vi "Startup.vi"(6 "LabVIEW Web Service":refnum<class "Web Service.lvclass">) -> ()   [LabVIEW 2014]
uses:
  <vilib>/wsapi/Web Service.lvclass
  Configuration/Global_Configurations.vi
panel:
  # "Use the web service input terminal to call the VIs on the Service subpalette of the Web Services palette. Do not remove it from the connector pane unless you don't need access to the palette."
  # "Any additional terminals added to the connector pane of a startup VI will be ignored."
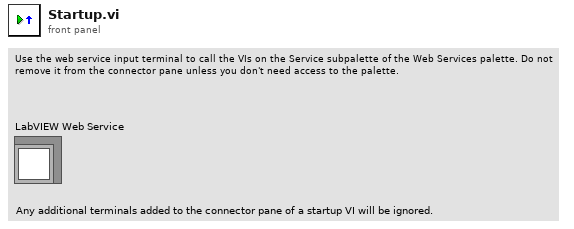
[diagram p1: front panel]
types:
  T1 = cluster{"Path":path, "Name":string, "Authors":string, "Keywords":string, "Description":string, "Cameras":cluster{"Base URL":string, "Path":string, "Name":string}[]}[]
  T2 = cluster{"Path":path, "Name":string, "Authors":string, "Keywords":string, "Description":string, "Cameras":cluster{"Base URL":string, "Path":string, "Name":string}[]}
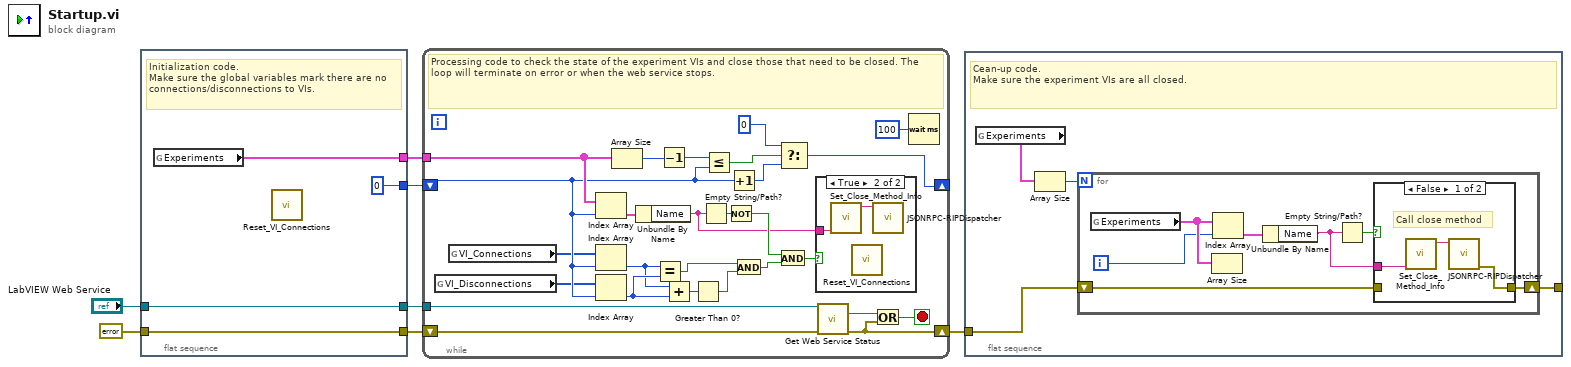
[diagram p0: block diagram]
diagram:
  n1 = flat-sequence {
    tunnel: "LabVIEW Web Service" -> [w11]
    tunnel: [w11] -> w6
    tunnel: [w10] -> w5
    tunnel: errorcluster {"status"=FALSE, "code"=0, "source"=""} ("error constant") -> [w10]
    tunnel: [0] -> w2
    tunnel: [w8] -> w1
    frame #0 {
      # "Initialization code.\nMake sure the global variables mark there are no connections/disconnections to VIs."
      n2 = global read "Global_Configurations.vi" "Experiments"() -> (w8:T1)
      n3 = call "Reset_VI_Connections.vi"() -> ()  [unwired: 12 in]
    }
  }
  n4 = while {
    tunnel: w6 -> [w37]
    shift-right: [w34] -> w3
    shift-left: w5 -> [w35]
    shift-right: [w25] -> _
    shift-left: w2 -> [w20]
    tunnel: w1 -> [w22]
    stop <- w36 stop-if-true
    # "Processing code to check the state of the experiment VIs and close those that need to be closed. The loop will terminate on error or when the web service stops."
    n5 = global read "Global_Configurations.vi" "VI_Disconnections"() -> (w14:u8[])
    n6 = global read "Global_Configurations.vi" "VI_Connections"() -> (w15:u8[])
    n7 = Index Array(array=w22, index=w20) -> (element=w29:T2)
    n8 = Index Array(array=w15, index=w20) -> (element=w12:u8)
    n9 = Index Array(array=w14, index=w20) -> (element=w13:u8)
    n10 = Array Size(array=w22) -> (size(s)=w28:i32)
    n11 = Unbundle By Name(w29) -> ("Name"=w21:string)
    n12 = Equal?(x=w12, y=w13) -> (x = y?=w18:bool)
    n13 = Decrement(x=w28) -> (x-1=w27:i32)
    n14 = Add(x=w12, y=w13) -> (x+y=w16:u8)
    n15 = Greater Than 0?(x=w16) -> (x > 0?=w17:bool)
    n16 = Empty String/Path?(string/path=w21) -> (empty?=w30:bool)
    n17 = Less Or Equal?(x=w27, y=w20) -> (x <= y?=w26:bool)
    n18 = Not(x=w30) -> (.not. x?=w31:bool)
    n19 = Increment(x=w20) -> (x+1=w23:i32)
    n20 = And(x=w18, y=w17) -> (x .and. y?=w19:bool)
    n21 = And(x=w31, y=w19) -> (x .and. y?=w32:bool)
    n22 = Select(t=0 ("f"), s=w26, f=w23) -> (s? t:f=w25:i32)
    n23 = case shown="True" w32 {
      tunnel: w21 -> [_ w39]
      frame False {
      }
      frame True {
        n24 = call "Set_Close_Method_Info.vi"("expId"=w39) -> ("String"=w40:string)  [unwired: 10 in]
        n25 = call "Reset_VI_Connections.vi"() -> ()  [unwired: 12 in]
        n26 = call "JSONRPC-RIPDispatcher.vi"("input string"=w40) -> ()  [unwired: 9 in, 2 out]
      }
    }
    n27 = call <vilib>:"Get Web Service Status.vi"("LabVIEW Web Service"=w37, "error in (no error)"=w35) -> ("service stopping?"=w38:bool, "error out"=w34:errorcluster)  [unwired: 11 in, 1 out]
    n28 = Or(x=w38, y=w34) -> (x .or. y?=w36:bool)
    n29 = Wait (ms)(milliseconds to wait=u32 100) -> ()  [unwired: 1 out]
  }
  n30 = flat-sequence {
    tunnel: w3 -> [w42]
    tunnel: [w41] -> _
    frame #0 {
      # "Cean-up code.\nMake sure the experiment VIs are all closed."
      n31 = global read "Global_Configurations.vi" "Experiments"() -> (w44:T1)
      n32 = Array Size(array=w44) -> (size(s)=w43:i32)
      n33 = for {
        N: w43 -> [_]
        shift-right: [w46] -> w41
        shift-left: w42 -> [w45]
        i -> [w49]
        n34 = global read "Global_Configurations.vi" "Experiments"() -> (w50:T1)
        n35 = Array Size(array=w50) -> ()  [unwired: 1 out]
        n36 = Index Array(array=w50, index=w49) -> (element=w51:T2)
        n37 = Unbundle By Name(w51) -> ("Name"=w47:string)
        n38 = Empty String/Path?(string/path=w47) -> (empty?=w48:bool)
        n39 = case shown="False" w48 {
          tunnel: w47 -> [w53 _]
          tunnel: [w52 w55] -> w46
          tunnel: w45 -> [_ w55]
          frame False {
            # "Call close method"
            n40 = call "Set_Close_Method_Info.vi"("expId"=w53) -> ("String"=w54:string)  [unwired: 10 in]
            n41 = call "JSONRPC-RIPDispatcher.vi"("input string"=w54) -> ("error out"=w52:errorcluster)  [unwired: 9 in, 1 out]
          }
          frame True {
          }
        }
      }
    }
  }
